vi "test_Receive - Monitor (Mulit Record).vi"() -> ()   [LabVIEW 2020]
doc: "Overview: Implements a Chronological Monitor for a specific Board and Port.\n\nRequirement: One AIM ARINC-664 board with installed AIM ARINC 664 BSP.\nRestrictions: None.\nInstruction:\n1. Select the Board ID (0 if you have only one board in your system).\n2. Run the VI.\n3. See the result in Current IRIG Time\nFor detailed information about functions use, see documents in <BSP Installation folder>\\AIM GmbH\\Arinc 664 Windows BSP <version>\\Doc."
uses:
  <instrlib>/AIM GmbH/_AIM 664/_controls/session_monitor_config.ctl
  Shared/Frame.ctl
  <instrlib>/AIM GmbH/_AIM 664/_controls/monitor_becw_type.ctl
  <instrlib>/AIM GmbH/_AIM 664/_controls/monitor_fhInfol_type.ctl
  <instrlib>/AIM GmbH/_AIM 664/_controls/monitor_entrySize_type.ctl
  <instrlib>/AIM GmbH/_AIM 664/_controls/monitor_fhw0_type.ctl
  <instrlib>/AIM GmbH/_AIM 664/_controls/monitor_fhw1_type.ctl
  <instrlib>/AIM GmbH/_AIM 664/bsp/Fdx Create Session (RX-Monitor).vi
  <instrlib>/AIM GmbH/_AIM 664/bsp/Fdx Start (Rx).vi
  <instrlib>/AIM GmbH/_AIM 664/bsp/Fdx Stop (Rx).vi
  <instrlib>/AIM GmbH/_AIM 664/AIM664LV.lvlib
panel:
  out "HeaderInfo":T1[](array[typedef]) {"FHW0"."MacID" format="%03b"}
  out "BECW":T5[](array[typedef])
  out "Payloads":T6[](array[typedef])
  out "FramesToRead":u32
  out "BytesToRead":u32
  out "BytesRead":u32
  out "Read data":bool
  out "EntryRead":u32
  out "Synchronized":u32
  out "QueueStatus":T7 {"QueueStatus" items=["FDX_MON_STAT_EMPTY", "FDX_MON_STAT_ FILLED", "FDX_MON_STAT_ FULL", "FDX_MON_STAT_ OVERFLOW", "FDX_MON_STAT_ ERROR"]}
  out "current irig time":T8={"SignOut"=40, "DayOut"=1, "HourOut"=1, "MinOut"=28, "SecondOut"=39, "MilliSecOut"=539, "MicroSecOut"=300, "NanoSecOut"=0, "InfoOut"=0, "Mode"=3}
  in  "fetch period ms":u32=100
  in  "MaxFileSize MB (1)":u32=1
  in  "MonCapMode":T9 {"Strobe" items=["FDX_MON_STROBE_DIS", "FDX_MON_STROBE_STOP", "FDX_MON_STROBE_START"]; "CaptureMode" items=["FDX_MON_SINGLE ", "FDX_MON_CONTINUOUS", "FDX_MON_SELECTIVE", "FDX_MON_RECORDING", "FDX_MON_REROS", "FDX_MON_HMU"]}
  out "PortInitOut":T10={"PortConfig"=0, "PortUsed"=1, "GlobalMemFree"=0, "SharedMemFree"=0} {"PortConfig" items=["FDX_SINGLE", "FDX_REDUNDANT"]}
  in  "Port":u32
  in  "Board":u32=1
  in  "MonitorConfig":T11={"DefaultCronoMode"=2, "GlbMonBufferSizeIn"=0} {"DefaultCronoMode" items=["FDX_RX_DEFAULT_ENA_CNT", "FDX_RX_DEFAULT_MON_ENA_ALL", "FDX_RX_DEFAULT_MON_ENA_GOOD"]}
  out "error out":errorcluster
  in  "stop":bool
  out "current time":timestamp
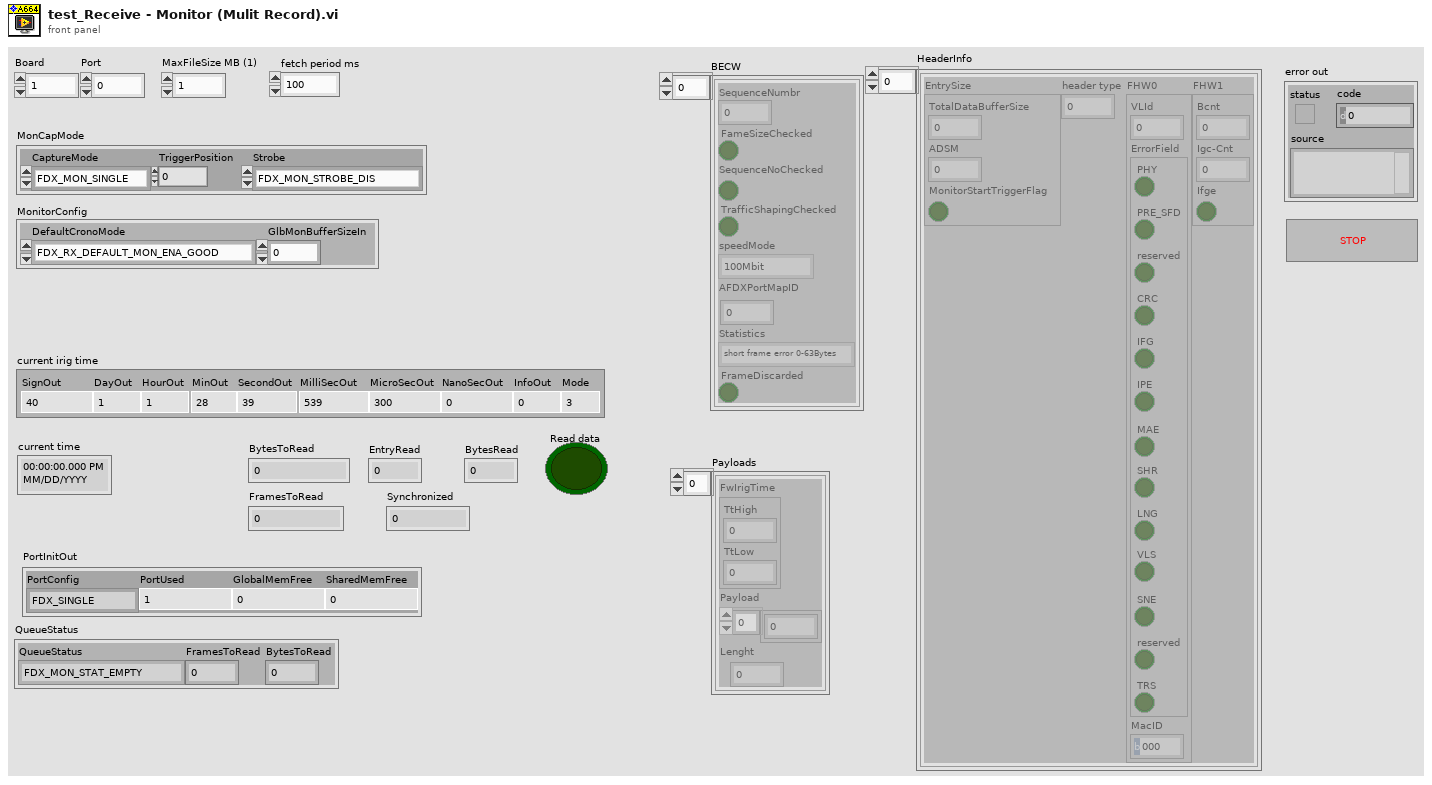
[diagram p1: front panel]
types:
  T1 = typedef "AIM664LV.lvlib/monitor_fhInfol_type.ctl" = cluster{"EntrySize":T2, "header type":u32, "FHW0":T3, "FHW1":T4}
  T2 = typedef "AIM664LV.lvlib/monitor_entrySize_type.ctl" = cluster{"TotalDataBufferSize":u16, "ADSM":u16, "MonitorStartTriggerFlag":bool}
  T3 = typedef "AIM664LV.lvlib/monitor_fhw0_type.ctl" = cluster{"VLId":u16, "ErrorField":cluster{"PHY":bool, "PRE_SFD":bool, "reserved":bool, "CRC":bool, "IFG":bool, "IPE":bool, "MAE":bool, "SHR":bool, "LNG":bool, "VLS":bool, "SNE":bool, "reserved":bool, "TRS":bool}, "MacID":u8}
  T4 = typedef "AIM664LV.lvlib/monitor_fhw1_type.ctl" = cluster{"Bcnt":u16, "Igc-Cnt":u16, "Ifge":bool}
  T5 = typedef "AIM664LV.lvlib/monitor_becw_type.ctl" = cluster{"SequenceNumbr":u8, "FameSizeChecked":bool, "SequenceNoChecked":bool, "TrafficShapingChecked":bool, "speedMode":enum16{"100Mbit", "10Mbit", "1Gbit"}, "AFDXPortMapID":u8, "Statistics":enum16{"short frame error 0-63Bytes", "64-127 Bytes", "128-255 Bytes", "256-511 Bytes", "512-1023 Bytes", "1024-1518 Bytes", ">1518 Bytes"}, "FrameDiscarded":bool}
  T6 = typedef "Frame.ctl" = cluster{"FwIrigTime":cluster{"TtHigh":u32, "TtLow":u32}, "Payload":u8[], "Lenght":u32}
  T7 = cluster{"QueueStatus":u32, "FramesToRead":u32, "BytesToRead":u32}
  T8 = cluster{"SignOut":i32, "DayOut":u32, "HourOut":u32, "MinOut":u32, "SecondOut":u32, "MilliSecOut":u32, "MicroSecOut":u32, "NanoSecOut":u32, "InfoOut":u32, "Mode":u32}
  T9 = cluster{"CaptureMode":u32, "TriggerPosition":u32, "Strobe":u32}
  T10 = cluster{"PortConfig":u32, "PortUsed":u32, "GlobalMemFree":u32, "SharedMemFree":u32}
  T11 = typedef "AIM664LV.lvlib/session_monitor_config.ctl" = cluster{"DefaultCronoMode":u32, "GlbMonBufferSizeIn":u32}
  T12 = cluster{"EntryRead":u32, "BytesRead":u32, "Synchronized":u32, "ReadBuffer":u8[]}
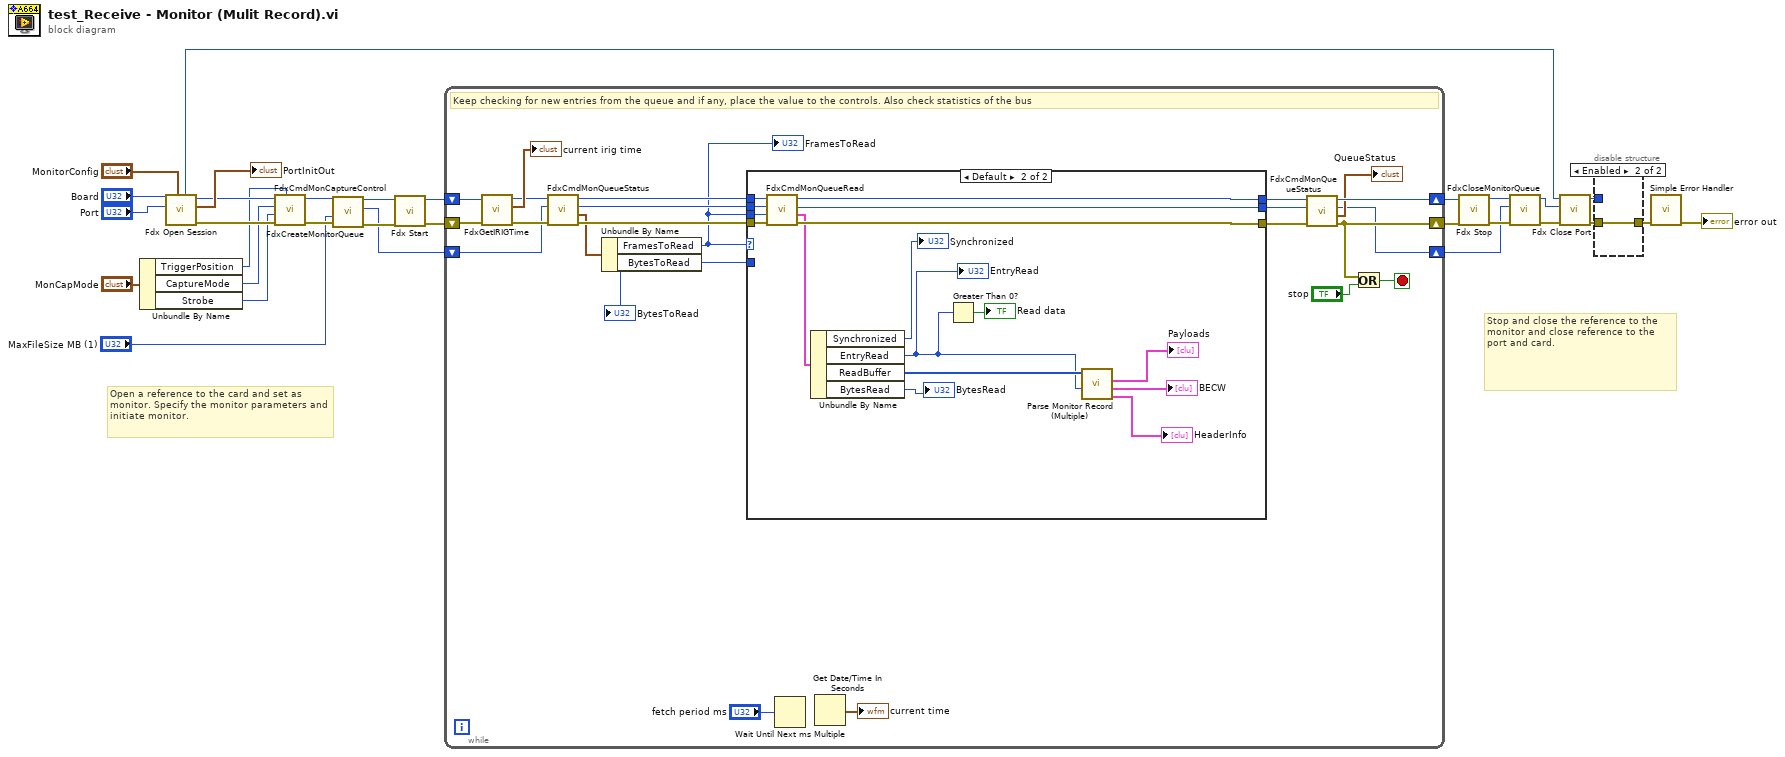
[diagram p0: block diagram]
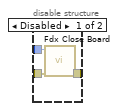
[diagram p3: hidden frame]
diagram:
  # "Stop and close the reference to the monitor and close reference to the port and card."
  # "Open a reference to the card and set as monitor. Specify the monitor parameters and initiate monitor."
  n1 = Unbundle By Name("MonCapMode") -> ("TriggerPosition"=w4:u32, "CaptureMode"=w3:u32, "Strobe"=w11:u32)
  n2 = call-poly <instrlib>:"Fdx Open Session.vi"("MonitorConfig"="MonitorConfig", "port"="Port", "board"="Board") -> ("error out"=w22:errorcluster, "PortInitOut"=→"PortInitOut":T10, "InstrumentHandle_port out"=w23:u32, "InstrumentHandle_board out"=w14:u32)  [unwired: 3 in, 2 out]
  n3 = call <instrlib>:"FdxCmdMonCaptureControl.vi"("TriggerPosition"=w4, "error in"=w22, "Strobe"=w11, "CaptureMode"=w3, "InstrumentHandle_port in"=w23) -> ("error out"=w21:errorcluster, "InstrumentHandle_port out"=w20:u32)  [unwired: 5 in]
  n4 = call <instrlib>:"FdxCreateMonitorQueue.vi"("error in (no error)"=w21, "MaxFileSize MB (1)"="MaxFileSize MB (1)", "InstrumentHandle_port in"=w20) -> ("error out"=w18:errorcluster, "QueueIdOut"=w17:u32, "InstrumentHandle_port out"=w19:u32)  [unwired: 5 in, 1 out]
  n5 = call-poly <instrlib>:"Fdx Start.vi"("error in"=w18, "InstrumentHandle_port in"=w19) -> ("error out"=w28:errorcluster, "InstrumentHandle_port out"=w30:u32)  [unwired: 8 in]
  n6 = while {
    shift-right: [w43] -> w29
    shift-left: w30 -> [w50]
    shift-right: [w44] -> w27
    shift-left: w28 -> [w49]
    shift-right: [w40] -> w8
    shift-left: w17 -> [w34]
    stop <- w51 stop-if-true
    # "Keep checking for new entries from the queue and if any, place the value to the controls. Also check statistics of the bus"
    n7 = call <instrlib>:"FdxGetIRIGTime.vi"("error in"=w49, "InstrumentHandle_board in"=w50) -> ("error out"=w39:errorcluster, "Curent Irig Time"=→"current irig time":T8, "InstrumentHandle_board out"=w38:u32)  [unwired: 7 in]
    n8 = call <instrlib>:"FdxCmdMonQueueStatus.vi"("error in"=w39, "QueueId"=w34, "InstrumentHandle_port"=w38) -> ("error out"=w37:errorcluster, "QueueStatus"=w35:T7, "QueueIdOut"=w33:u32, "InstrumentHandle_port"=w36:u32)  [unwired: 5 in]
    n9 = Unbundle By Name(w35) -> ("FramesToRead"=w32:u32, "BytesToRead"=w31:u32)
    "BytesToRead" <- w31
    "FramesToRead" <- w32
    n10 = case shown="Default" w32 {
      tunnel: [w56 w72] -> w46
      tunnel: [w54 w71] -> w45
      tunnel: [w55 w70] -> w41
      tunnel: w37 -> [w54 w69]
      tunnel: w36 -> [w56 w68]
      tunnel: w33 -> [w55 w67]
      tunnel: w32 -> [_ w62]
      tunnel: w31 -> [_ _]
      frame 0 {
      }
      frame Default {
        n11 = call <instrlib>:"FdxCmdMonQueueRead.vi"("error in"=w69, "EntryCount"=w62, "QueueId"=w67, "InstrumentHandle_port"=w68) -> ("error out"=w71:errorcluster, "QueueReadOut"=w65:T12, "QueueIdOut"=w70:u32, "InstrumentHandle_port"=w72:u32)  [unwired: 4 in]
        n12 = Unbundle By Name(w65) -> ("Synchronized"=→"Synchronized":u32, "EntryRead"=w60:u32, "ReadBuffer"=w61:u8[], "BytesRead"=→"BytesRead":u32)
        "EntryRead" <- w60
        n13 = Greater Than 0?(x=w60) -> (x > 0?=→"Read data":bool)
        n14 = call <instrlib>:"Parse Monitor Record (Multiple).vi"("record count"=w60, "Record In"=w61) -> ("HeaderInfo"=→"HeaderInfo":T1[], "BECW"=→"BECW":T5[], "Payloads"=→"Payloads":T6[])  [unwired: 6 in, 1 out]
      }
    }
    n15 = Wait Until Next ms Multiple(millisecond multiple="fetch period ms") -> ()  [unwired: 1 out]
    n16 = Get Date/Time In Seconds() -> (seconds since 1Jan1904=→"current time":timestamp)
    n17 = call <instrlib>:"FdxCmdMonQueueStatus.vi"("error in"=w45, "QueueId"=w41, "InstrumentHandle_port"=w46) -> ("error out"=w44:errorcluster, "QueueStatus"=→"QueueStatus":T7, "QueueIdOut"=w40:u32, "InstrumentHandle_port"=w43:u32)  [unwired: 5 in]
    n18 = Or(x=w44, y="stop") -> (x .or. y?=w51:bool)
  }
  n19 = call-poly <instrlib>:"Fdx Stop.vi"("error in"=w27, "InstrumentHandle_port in"=w29) -> ("error out"=w16:errorcluster, "InstrumentHandle_port out"=w10:u32)  [unwired: 8 in]
  n20 = call <instrlib>:"FdxCloseMonitorQueue.vi"("error in"=w16, "QueueId"=w8, "InstrumentHandle_port in"=w10) -> ("error out"=w15:errorcluster, "InstrumentHandle_port out"=w9:u32)  [unwired: 7 in]
  n21 = call <instrlib>:"Fdx Close Port.vi"("error in"=w15, "InstrumentHandle_port in"=w9, "InstrumentHandle_board in"=w14) -> ("error out"=w6:errorcluster, "InstrumentHandle_board out"=w1:u32)  [unwired: 7 in]
  n22 = disable-structure shown="Enabled" {
    disable-tunnel: w6 -> [w75 w76]
    disable-tunnel: [w74 w76] -> w2
    disable-tunnel: w1 -> [w73 _]
    frame Disabled {
      n23 = call <instrlib>:"Fdx Close Board.vi"("error in"=w75, "InstrumentHandle_board in"=w73) -> ("error out"=w74:errorcluster)  [unwired: 9 in]
    }
    frame Enabled {
    }
  }
  n24 = call <vilib>:"Simple Error Handler.vi"("error in (no error)"=w2) -> ("error out"=→"error out":errorcluster)  [unwired: 4 in, 4 out]
